vi "SVFA Unit Conversion (Waterfall).vi"(0 "waterfall":T2, 1 "desired scaling":T9 {"dB reference (0: no change)" format="%.2f"}, 2 "spectral density desired":T1(ring), 4 "spectrum info in":T3={"channel name"="", "description"="", "x-axis units"=0, "spectral info"={"spectrum type"=enum."Power [Magnitude^2]", "linear/dB"=enum."linear", "window"=0, "window size"=0, "FFT size"=0}, "engineering units"=0, "custom label"="", "dB reference [EU]"=0.0, "peak units"=enum."rms", "weighting filter"=0, "spectral density?"=FALSE, "unit label"="", "spectrum skewed?"=FALSE, "complimentary spectrum units"=enum."none"} {"x-axis units" items=["Time (s)"=0, "Frequency-CB (Hz)"=1, "Frequency-CPB (Hz)"=1248, "Frequency-Arbitrary (Hz)"=2357, "Quefrency (s)"=2, "Revolutions (rev)"=3, "Order"=4, "Speed (RPM)"=11, "Speed (rad/s)"=21, "Index"=65535]; "weighting filter" items=["Linear", "A-weighting", "B-weighting", "C-weighting", "ITU-R 468-4", "Dolby", "CCITT", "C-message", "Wb", "Wc", "Wd", "We", "Wf", "Wh", "Wj", "Wk", "Wm", "AES17 20 kHz lowpass", "AES17 40 kHz lowpass", "AES17 20 kHz highpass", "AES17 40 kHz highpass"]; "dB reference [EU]" format="%.2f"; "engineering units" items=["custom..."=0, "V"=1, "A"=21, "C"=30, "pC"=31, "s"=32, "-"=29, "Pa"=2, "N"=20, "g"=3, "m/s^2"=4, "m/s"=5, "m"=6, "mm/s"=12, "mm"=13, "micron/s"=14, "micron"=15, "in/s^2"=7, "in/s"=8, "in"=9, "mil/s"=10, "mil"=11, "rad/s^2"=16, "rad/s"=17, "rad"=18, "deg/s^2"=26, "deg/s"=27, "deg"=28, "RPM"=22, "cycle/s^2"=23, "Hz"=24, "cycle"=25, "strain"=19]; "spectral info"."window" items=["None "=0, "Hanning"=1, "Hamming"=2, "Blackman-Harris"=3, "Exact Blackman"=4, "Blackman"=5, "Flat Top"=6, "4 Term B-Harris "=7, "7 Term B-Harris"=8, "Low Sidelobe"=9, "Force - Exponential"=10, "Gaussian"=62]}, 5 "error in (no error)":errorcluster) -> (14 "converted waterfall":T2, 15 "unit label":string, 18 "spectrum info out":T3={"channel name"="", "description"="", "x-axis units"=0, "spectral info"={"spectrum type"=enum."Power [Magnitude^2]", "linear/dB"=enum."linear", "window"=0, "window size"=0, "FFT size"=0}, "engineering units"=0, "custom label"="", "dB reference [EU]"=0.0, "peak units"=enum."rms", "weighting filter"=0, "spectral density?"=FALSE, "unit label"="", "spectrum skewed?"=FALSE, "complimentary spectrum units"=enum."none"} {"x-axis units" items=["Time (s)"=0, "Frequency-CB (Hz)"=1, "Frequency-CPB (Hz)"=1248, "Frequency-Arbitrary (Hz)"=2357, "Quefrency (s)"=2, "Revolutions (rev)"=3, "Order"=4, "Speed (RPM)"=11, "Speed (rad/s)"=21, "Index"=65535]; "weighting filter" items=["Linear", "A-weighting", "B-weighting", "C-weighting", "ITU-R 468-4", "Dolby", "CCITT", "C-message", "Wb", "Wc", "Wd", "We", "Wf", "Wh", "Wj", "Wk", "Wm", "AES17 20 kHz lowpass", "AES17 40 kHz lowpass", "AES17 20 kHz highpass", "AES17 40 kHz highpass"]; "dB reference [EU]" format="%.2f"; "engineering units" items=["custom..."=0, "V"=1, "A"=21, "C"=30, "pC"=31, "s"=32, "-"=29, "Pa"=2, "N"=20, "g"=3, "m/s^2"=4, "m/s"=5, "m"=6, "mm/s"=12, "mm"=13, "micron/s"=14, "micron"=15, "in/s^2"=7, "in/s"=8, "in"=9, "mil/s"=10, "mil"=11, "rad/s^2"=16, "rad/s"=17, "rad"=18, "deg/s^2"=26, "deg/s"=27, "deg"=28, "RPM"=22, "cycle/s^2"=23, "Hz"=24, "cycle"=25, "strain"=19]; "spectral info"."window" items=["None "=0, "Hanning"=1, "Hamming"=2, "Blackman-Harris"=3, "Exact Blackman"=4, "Blackman"=5, "Flat Top"=6, "4 Term B-Harris "=7, "7 Term B-Harris"=8, "Low Sidelobe"=9, "Force - Exponential"=10, "Gaussian"=62]}, 19 "error out":errorcluster)   [LabVIEW 2017]
doc: "Converts between dB/linear, magnitude/magnitude^2, rms/peak/peak-peak, spectrum/spectral density, and dB ref1/dB ref2. Wire data to the <B>spectrum</B> input to determine the polymorphic instance to use or manually select the instance."
uses:
  <vilib>/addons/_NISVFA/_Shared subVIs/Controls/svc_Spectrum Info.ctl
  <vilib>/addons/_NISVFA/_Shared subVIs/Controls/svc_X-Axis Units.ctl
  <vilib>/addons/_NISVFA/_Shared subVIs/Controls/svc_Spectrum Type.ctl
  <vilib>/addons/_NISVFA/_Shared subVIs/Controls/svc_Engineering Units Text Ring.ctl
  <vilib>/addons/_NISVFA/_Shared subVIs/Controls/svc_Weighting Filter Text Ring.ctl
  <vilib>/addons/_NISVFA/_Shared subVIs/Controls/svc_Complimentary Spectrum Units.ctl
  <vilib>/addons/_NISVFA/_Spectrum Processing/subVIs/svfa_Conversion Utility (spectrum info).vi
  <vilib>/addons/_NISVFA/_Spectrum Processing/subVIs/svfa_Peak to RMS to Peak2Peak.vi
  <vilib>/addons/_NISVFA/_Spectrum Processing/subVIs/svfa_Mag to Mag2.vi
  <vilib>/addons/_NISVFA/_Spectrum Processing/subVIs/svfa_Linear to dB.vi
  <vilib>/addons/_NISVFA/_Spectrum Processing/subVIs/svfa_dBrefA to dBrefB.vi
  <vilib>/addons/_NISVFA/_Spectrum Processing/subVIs/svfa_Spectrum to Spectral Density.vi
  <vilib>/addons/_NISVFA/_Shared subVIs/Common/svc_Get Weighting Enum and Labels.vi
  <vilib>/addons/_NISVFA/_Shared subVIs/Common/svc_Unit Label Lexical Class.vi
  <vilib>/addons/_NISVFA/_Shared subVIs/Common/svc_Engineering Units to Unit Label.vi
  <vilib>/addons/_NISVFA/_Shared subVIs/Common/svc_Format Value (DBL).vi
  <vilib>/addons/_NISVFA/_Shared subVIs/Common/svc_Window Parameters.vi
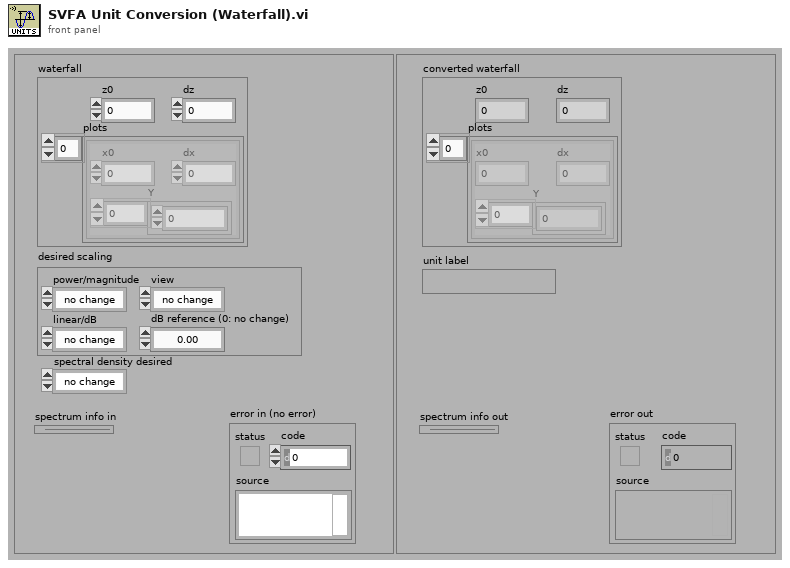
[diagram p1: front panel]
types:
  T1 = enum16{"no change", "spectrum", "spectral density"}
  T2 = cluster{"z0":dbl, "dz":dbl, "plots":cluster{"x0":dbl, "dx":dbl, "Y":dbl[]}[]}
  T3 = typedef "svc_Spectrum Info.ctl" = cluster{"channel name":string, "description":string, "x-axis units":T4, "spectral info":cluster{"spectrum type":T5, "linear/dB":enum16{"linear", "dB"}, "window":u16, "window size":i32, "FFT size":i32}, "engineering units":T6, "custom label":string, "dB reference [EU]":dbl, "peak units":enum16{"rms", "peak", "peak-peak"}, "weighting filter":T7, "spectral density?":bool, "unit label":string, "spectrum skewed?":bool, "complimentary spectrum units":T8}
  T4 = typedef "svc_X-Axis Units.ctl" = u16
  T5 = typedef "svc_Spectrum Type.ctl" = enum16{"FFT Spectrum [complex]", "Amplitude [Magnitude]", "Power [Magnitude^2]", "Cross Spectrum [complex]", "Frequency Response [Complex]"}
  T6 = typedef "svc_Engineering Units Text Ring.ctl" = u16
  T7 = typedef "svc_Weighting Filter Text Ring.ctl" = u16
  T8 = typedef "svc_Complimentary Spectrum Units.ctl" = enum16{"none", "radians", "degrees", "cycles", "imaginary"}
  T9 = cluster{"linear/dB":enum16{"no change", "linear", "dB"}, "dB reference (0: no change)":dbl, "power/magnitude":enum16{"no change", "power", "magnitude"}, "view":enum16{"no change", "rms", "peak", "peak-peak"}}
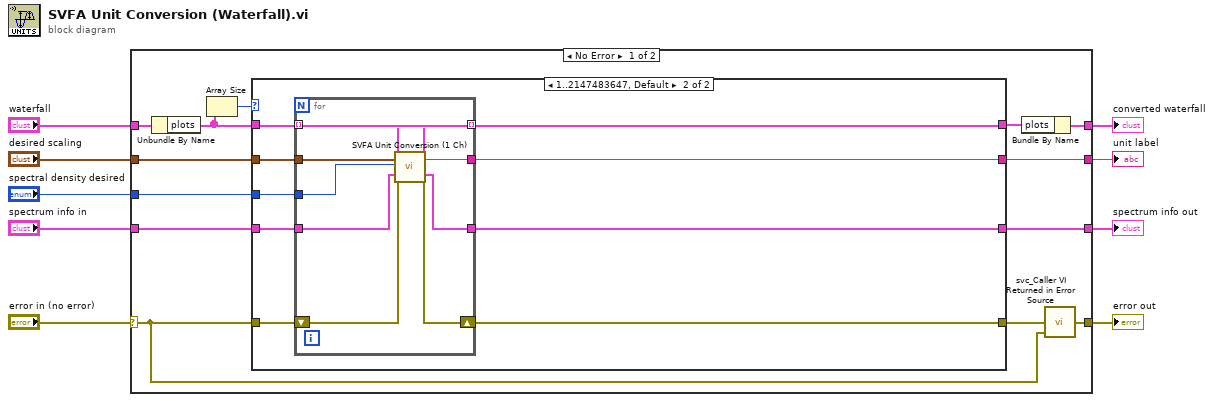
[diagram p0: block diagram]
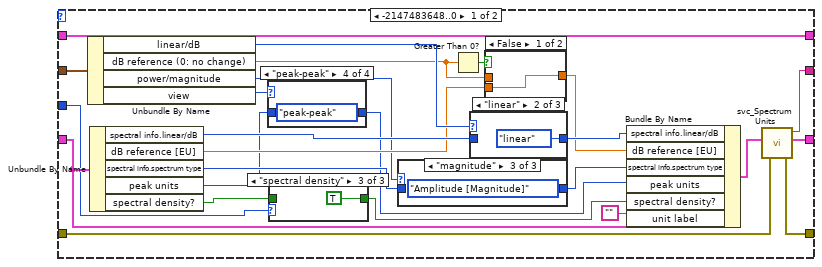
[diagram p2: hidden frame]
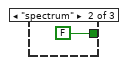
[diagram p4: hidden frame]
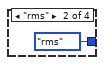
[diagram p6: hidden frame]
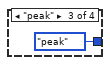
[diagram p7: hidden frame]
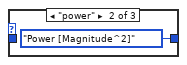
[diagram p9: hidden frame]
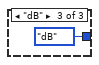
[diagram p12: hidden frame]
diagram:
  n1 = case shown="No Error" "error in (no error)" {
    selector: "error in (no error)" -> [w14 w83]
    tunnel: "spectrum info in" -> [w22 w82]
    tunnel: "waterfall" -> [w13 w81]
    tunnel: "desired scaling" -> [w21 _]
    tunnel: [w16 w83] -> w6
    tunnel: [w12 w81] -> w5
    tunnel: [w18 w82] -> w4
    tunnel: [w17 _] -> w3
    tunnel: "spectral density desired" -> [w15 _]
    frame No Error {
      n2 = Unbundle By Name(w13) -> ("plots"=w11:cluster{"x0":dbl, "dx":dbl, "Y":dbl[]}[])
      n3 = Array Size(array=w11) -> (size(s)=w10:i32)
      n4 = case shown="1..2147483647, Default" w10 {
        tunnel: w22 -> [w39 w71]
        tunnel: w21 -> [w46 w70]
        tunnel: [w44 w69] -> w20
        tunnel: [w47 w68] -> w19
        tunnel: [w43 w67] -> w18
        tunnel: [w40 w66] -> w17
        tunnel: w15 -> [w25 w65]
        tunnel: w14 -> [w45 w64]
        tunnel: w11 -> [w47 w63]
        frame -2147483648..0 {
          n5 = Unbundle By Name(w46) -> ("linear/dB"=w38:enum16{"no change", "linear", "dB"}, "dB reference (0: no change)"=w34:dbl, "power/magnitude"=w31:enum16{"no change", "power", "magnitude"}, "view"=w28:enum16{"no change", "rms", "peak", "peak-peak"})
          n6 = Unbundle By Name(w39) -> ("spectral info.linear/dB"=w37:enum16{"linear", "dB"}, "dB reference [EU]"=w32:dbl, "spectral info.spectrum type"=w30:T5, "peak units"=w27:enum16{"rms", "peak", "peak-peak"}, "spectral density?"=w24:bool)
          n7 = case shown="\"peak-peak\"" w28 {
            tunnel: w27 -> [w51 _ _ _]
            tunnel: [w51 enum16{"rms", "peak", "peak-peak"}."rms" ("peak units") enum16{"rms", "peak", "peak-peak"}."peak" ("peak units") enum16{"rms", "peak", "peak-peak"}."peak-peak" ("peak units")] -> w26
            frame "no change", Default {
            }
            frame "rms" {
            }
            frame "peak" {
            }
            frame "peak-peak" {
            }
          }
          n8 = case shown="\"spectral density\"" w25 {
            tunnel: w24 -> [w48 _ _]
            tunnel: [w48 FALSE ("spectral density?") TRUE ("spectral density?")] -> w23
            frame "no change", Default {
            }
            frame "spectrum" {
            }
            frame "spectral density" {
            }
          }
          n9 = case shown="\"magnitude\"" w31 {
            tunnel: w30 -> [w55 _ _]
            tunnel: [w55 svc_Spectrum_Type."Power [Magnitude^2]" ("spectrum type") svc_Spectrum_Type."Amplitude [Magnitude]" ("spectrum type")] -> w29
            frame "no change", Default {
            }
            frame "power" {
            }
            frame "magnitude" {
            }
          }
          n10 = Greater Than 0?(x=w34) -> (x > 0?=w35:bool)
          n11 = case shown="\"linear\"" w38 {
            tunnel: w37 -> [w60 _ _]
            tunnel: [w60 enum16{"linear", "dB"}."linear" ("linear/dB") enum16{"linear", "dB"}."dB" ("linear/dB")] -> w36
            frame "no change", Default {
            }
            frame "linear" {
            }
            frame "dB" {
            }
          }
          n12 = case shown="False" w35 {
            tunnel: w34 -> [_ w59]
            tunnel: [w58 w59] -> w33
            tunnel: w32 -> [w58 _]
            frame False {
            }
            frame True {
            }
          }
          n13 = Bundle By Name(cluster=w39, "spectral info.linear/dB"=w36, "dB reference [EU]"=w33, "spectral info.spectrum type"=w29, "peak units"=w26, "spectral density?"=w23, "unit label"="") -> (w41:T3)
          n14 = call <vilib>:"svc_Spectrum Units.vi"("error in (no error)"=w45, "spectrum info in"=w41) -> ("error out"=w44:errorcluster, "spectrum info out"=w43:T3, "unit label"=w40:string)  [unwired: 2 in, 1 out]
        }
        frame 1..2147483647, Default {
          n15 = for {
            tunnel: [w80] -> w68 mode=indexing
            shift-right: [w79] -> w69
            shift-left: w64 -> [w78]
            tunnel: w63 -> [w77] mode=indexing
            tunnel: w70 -> [w76]
            tunnel: [w73] -> w66
            tunnel: w65 -> [w72]
            tunnel: w71 -> [w75]
            tunnel: [w74] -> w67
            n16 = call <vilib>:"SVFA Unit Conversion (1 Ch).vi"("spectrum"=w77, "desired scaling"=w76, "spectral density desired"=w72, "spectrum info in"=w75, "error in (no error)"=w78) -> ("converted spectrum"=w80:cluster{"x0":dbl, "dx":dbl, "magnitude":dbl[]}, "unit label"=w73:string, "spectrum info out"=w74:T3, "error out"=w79:errorcluster)  [unwired: 11 in]
          }
        }
      }
      n17 = Bundle By Name(cluster=w13, "plots"=w19) -> (w12:T2)
      n18 = call <vilib>:"svc_Caller VI Returned in Error Source.vi"("warning input to caller"=w14, "error in (no error)"=w20) -> ("error out"=w16:errorcluster)  [unwired: 3 in]
    }
    frame Error {
    }
  }
  "error out" <- w6
  "spectrum info out" <- w4
  "converted waterfall" <- w5
  "unit label" <- w3
